vi "beep_.vi"(0 "Signal Type":i32(ring) items=["Sine", "Multi-tone", "Square", "Triangular", "Saw-tooth", "Random", "Chirp"], 1 "MT Amplitude":dbl[](array[numeric]), 2 "MT Phase":dbl[](array[numeric]), 3 "Lowest Frequency":dbl, 5 "Freqency Range":i32(ring)=4000 items=["500 Hz"=500, "1 kHz"=1000, "2 kHz"=2000, "4 kHz"=4000, "8 kHz"=8000, "16 kHz"=16000], 7 "Block Size":i32(ring)=4096 items=["128"=128, "256 "=256, "500"=512, "1024"=1024, "2048"=2048, "4096"=4096, "8192"=8192, "16384"=16384], 9 "Amplitude":dbl=10.0, 11 "Frequency":dbl=1000.0, 12 "MT Frequency":dbl[](array[numeric]), 13 "duty cycle (%)":dbl=50.0 format="%0.2f", 14 "Highest Frequency":dbl, 15 "volume":dbl=100.0) -> (4 "Output":dbl[](array[numeric]))   [LabVIEW 2022 SP3]
uses:
  <vilib>/sound2/lvsound2.llb/Sound Output Task ID.ctl
  <vilib>/sound2/lvsound2.llb/Sound Output Set Volume (Single).vi
  <vilib>/sound2/lvsound2.llb/Sound Output Write (DBL Single).vi
  <vilib>/Analysis/NI_AALBase.lvlib
panel:
  out "Waveform Chart":dbl[](graph)
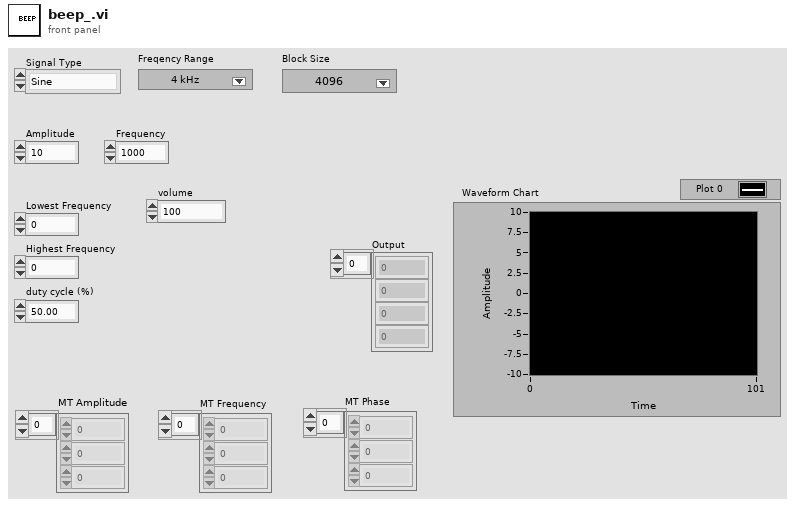
[diagram p1: front panel]
types:
  T1 = typedef "Sound Output Task ID.ctl" = u32
  T2 = cluster{"Numeric":dbl, "Numeric":dbl, "Numeric":dbl}
  T3 = cluster{"Numeric":dbl, "Numeric":dbl, "Numeric":dbl}[]
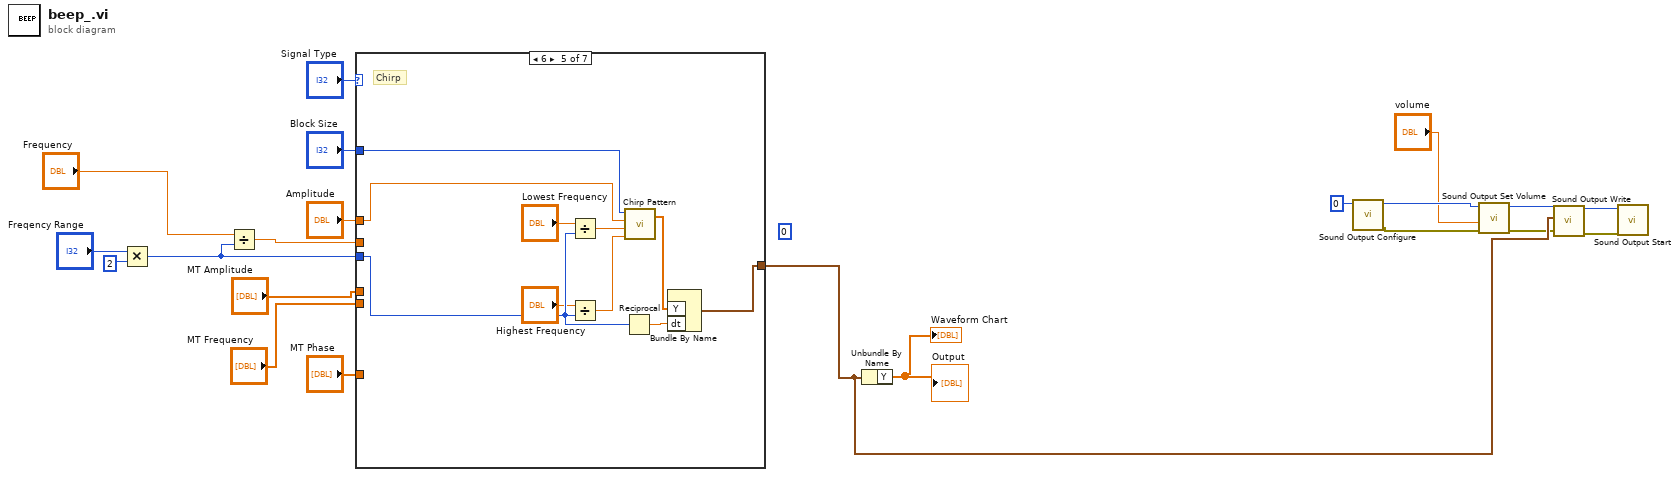
[diagram p0: block diagram]
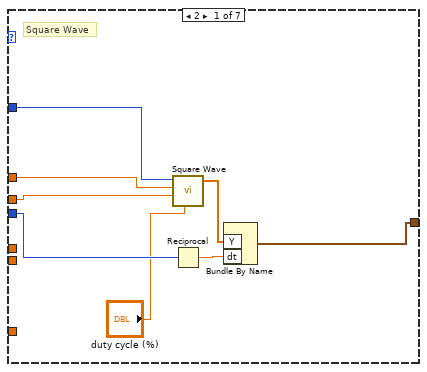
[diagram p2: hidden frame]
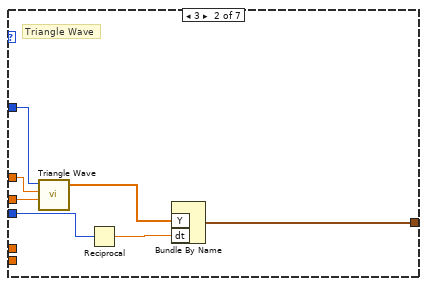
[diagram p3: hidden frame]
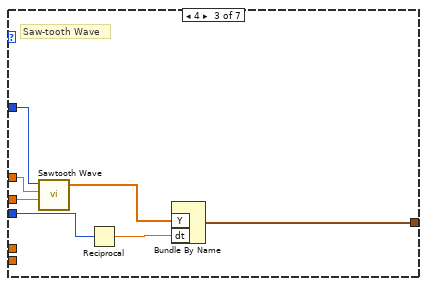
[diagram p4: hidden frame]
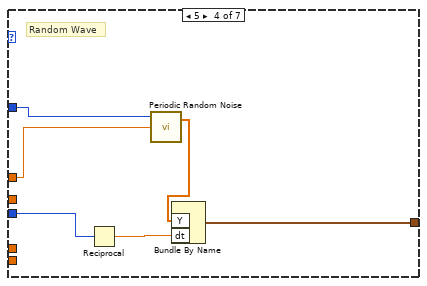
[diagram p5: hidden frame]
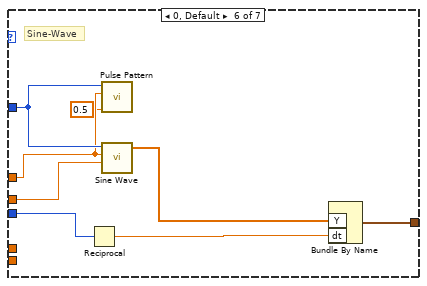
[diagram p6: hidden frame]
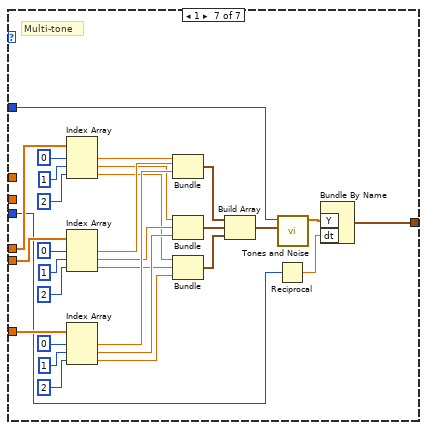
[diagram p7: hidden frame]
diagram:
  (unwired) T1 0 ("task ID")
  n1 = Multiply(x="Freqency Range", y=2) -> (x*y=w9:i32)
  n2 = Divide(x="Frequency", y=w9) -> (x/y=w14:dbl)
  n3 = case shown="6" "Signal Type" {
    tunnel: "Amplitude" -> [w26 w35 w42 w45 w56 w62 _]
    tunnel: "Block Size" -> [w28 w36 w43 w46 w55 w63 w97]
    tunnel: w14 -> [w24 w30 w41 _ _ w67 _]
    tunnel: w9 -> [w27 w32 w37 w47 w54 w66 w68]
    tunnel: [w25 w31 w38 w48 w57 w64 w94] -> w20
    tunnel: "MT Amplitude" -> [_ _ _ _ _ _ w92]
    tunnel: "MT Frequency" -> [_ _ _ _ _ _ w91]
    tunnel: "MT Phase" -> [_ _ _ _ _ _ w90]
    frame 2 {
      # "Square Wave"
      n4 = call <vilib>:"Square Wave.vi"("samples"=w28, "amplitude"=w26, "frequency"=w24, "duty cycle (%)"="duty cycle (%)") -> ("square wave"=w22:dbl[])  [unwired: 2 in, 2 out]
      n5 = Reciprocal(x=w27) -> (1/x=w29:dbl)
      n6 = Bundle By Name("Y"=w22, "dt"=w29) -> (w25:waveform(dbl))  [unwired: 1 in]
    }
    frame 3 {
      # "Triangle Wave"
      n7 = call <vilib>:"Triangle Wave.vi"("samples"=w36, "amplitude"=w35, "frequency"=w30) -> ("triangle wave"=w33:dbl[])  [unwired: 2 in, 2 out]
      n8 = Reciprocal(x=w32) -> (1/x=w34:dbl)
      n9 = Bundle By Name("Y"=w33, "dt"=w34) -> (w31:waveform(dbl))  [unwired: 1 in]
    }
    frame 4 {
      # "Saw-tooth Wave"
      n10 = call <vilib>:"Sawtooth Wave.vi"("samples"=w43, "amplitude"=w42, "frequency"=w41) -> ("sawtooth wave"=w39:dbl[])  [unwired: 2 in, 2 out]
      n11 = Reciprocal(x=w37) -> (1/x=w40:dbl)
      n12 = Bundle By Name("Y"=w39, "dt"=w40) -> (w38:waveform(dbl))  [unwired: 1 in]
    }
    frame 5 {
      # "Random Wave"
      n13 = Reciprocal(x=w47) -> (1/x=w49:dbl)
      n14 = call <vilib>:"Periodic Random Noise.vi"("spectral amplitude"=w45, "samples"=w46) -> ("periodic random noise"=w44:dbl[])  [unwired: 1 in, 1 out]
      n15 = Bundle By Name("Y"=w44, "dt"=w49) -> (w48:waveform(dbl))  [unwired: 1 in]
    }
    frame 6 {
      # "Chirp"
      n16 = Divide(x="Lowest Frequency", y=w54) -> (x/y=w52:dbl)
      n17 = Divide(x="Highest Frequency", y=w54) -> (x/y=w53:dbl)
      n18 = Reciprocal(x=w54) -> (1/x=w59:dbl)
      n19 = call <vilib>:"Chirp Pattern.vi"("f2"=w53, "f1"=w52, "amplitude"=w56, "samples"=w55) -> ("Chirp Pattern"=w58:dbl[])  [unwired: 1 out]
      n20 = Bundle By Name("Y"=w58, "dt"=w59) -> (w57:waveform(dbl))  [unwired: 1 in]
    }
    frame 0, Default {
      # "Sine-Wave"
      n21 = Reciprocal(x=w66) -> (1/x=w65:dbl)
      n22 = call <vilib>:"Pulse Pattern.vi"("width"=0.5, "amplitude"=w62, "samples"=w63) -> ()  [unwired: 1 in, 2 out]
      n23 = call <vilib>:"Sine Wave.vi"("samples"=w63, "amplitude"=w62, "frequency"=w67) -> ("sine wave"=w60:dbl[])  [unwired: 2 in, 2 out]
      n24 = Bundle By Name("Y"=w60, "dt"=w65) -> (w64:waveform(dbl))  [unwired: 1 in]
    }
    frame 1 {
      # "Multi-tone"
      n25 = Index Array(array=w92, index #1=0 ("index"), index #2=1 ("index"), index #3=2 ("index")) -> (element #1=w81:dbl, element #2=w78:dbl, element #3=w75:dbl)
      n26 = Index Array(array=w91, index #1=0 ("index"), index #2=1 ("index"), index #3=2 ("index")) -> (element #1=w80:dbl, element #2=w77:dbl, element #3=w74:dbl)
      n27 = Index Array(array=w90, index #1=0 ("index"), index #2=1 ("index"), index #3=2 ("index")) -> (element #1=w79:dbl, element #2=w76:dbl, element #3=w73:dbl)
      n28 = Bundle("Numeric"=w81, "Numeric"=w80, "Numeric"=w79) -> (w72:T2)  [unwired: 1 in]
      n29 = Bundle("Numeric"=w78, "Numeric"=w77, "Numeric"=w76) -> (w71:T2)  [unwired: 1 in]
      n30 = Bundle("Numeric"=w75, "Numeric"=w74, "Numeric"=w73) -> (w70:T2)  [unwired: 1 in]
      n31 = Build Array(w72, w71, w70) -> (w69:T3)
      n32 = Reciprocal(x=w68) -> (1/x=w96:dbl)
      n33 = call <vilib>:"Tones and Noise.vi"("tones"=w69, "samples"=w97) -> ("tones and noise"=w95:dbl[])  [unwired: 8 in, 1 out]
      n34 = Bundle By Name("Y"=w95, "dt"=w96) -> (w94:waveform(dbl))  [unwired: 1 in]
    }
  }
  n35 = Unbundle By Name(w20) -> ("Y"=→"Output" →"Waveform Chart":dbl[])
  n36 = call <vilib>:"Sound Output Configure.vi"("device ID"=u32 0) -> ("error out"=w2:errorcluster, "task ID"=w17:T1)  [unwired: 9 in]
  n37 = call-poly <vilib>:"Sound Output Set Volume.vi"("error in (no error)"=w2, "volume"="volume", "task ID"=w17) -> ("error out"=w19:errorcluster, "task ID out"=w21:T1)  [unwired: 7 in]
  n38 = call-poly <vilib>:"Sound Output Write.vi"("error in (no error)"=w19, "data"=w20, "task ID"=w21) -> ("error out"=w3:errorcluster, "task ID out"=w4:T1)  [unwired: 7 in]
  n39 = call <vilib>:"Sound Output Start.vi"("error in (no error)"=w3, "task ID"=w4) -> ()  [unwired: 8 in, 2 out]
